vi "read RS485 subVI.vi"(8 "error in (no error)":errorcluster, 11 "VISA Refnum in":refnum<visa-resource-name>="COM5") -> (0 "error out":errorcluster, 3 "DUT Config Data":T1)   [LabVIEW 2016]
uses:
  DUT Config Data ClusterType Def.ctl
  Control 2.ctl
  <vilib>/Instr/_visa.llb/VISA Configure Serial Port (Instr).vi
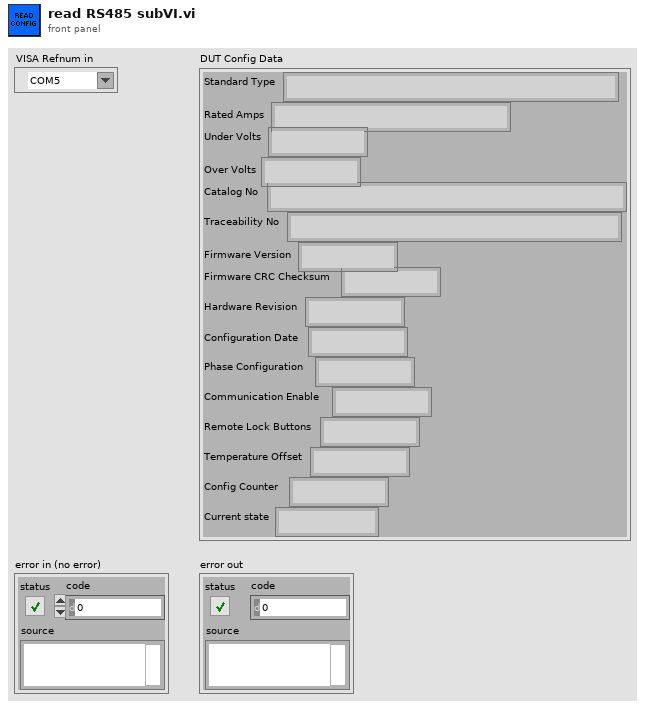
[diagram p1: front panel]
types:
  T1 = typedef "DUT Config Data ClusterType Def.ctl" = cluster{"Standard Type":string, "Rated Amps":string, "Under Volts":string, "Over Volts":string, "Catalog No":string, "Traceability No":string, "Firmware Version":string, "Firmware CRC Checksum":string, "Hardware Revision":string, "Configuration Date":string, "Phase Configuration":string, "Communication Enable":string, "Remote Lock Buttons":string, "Temperature Offset":string, "Config Counter":string, "Current state":string}
  T2 = typedef "Control 2.ctl" = enum16{"Message", "Write Config", "Read Config", "Listen"}
  T3 = cluster{"[0]":string, "[1]":string, "[2]":string, "[3]":string, "[4]":string, "[5]":string, "[6]":string, "[7]":string, "[8]":string, "[9]":string, "[10]":string, "[11]":string, "[12]":string, "[13]":string, "[14]":string, "[15]":string}
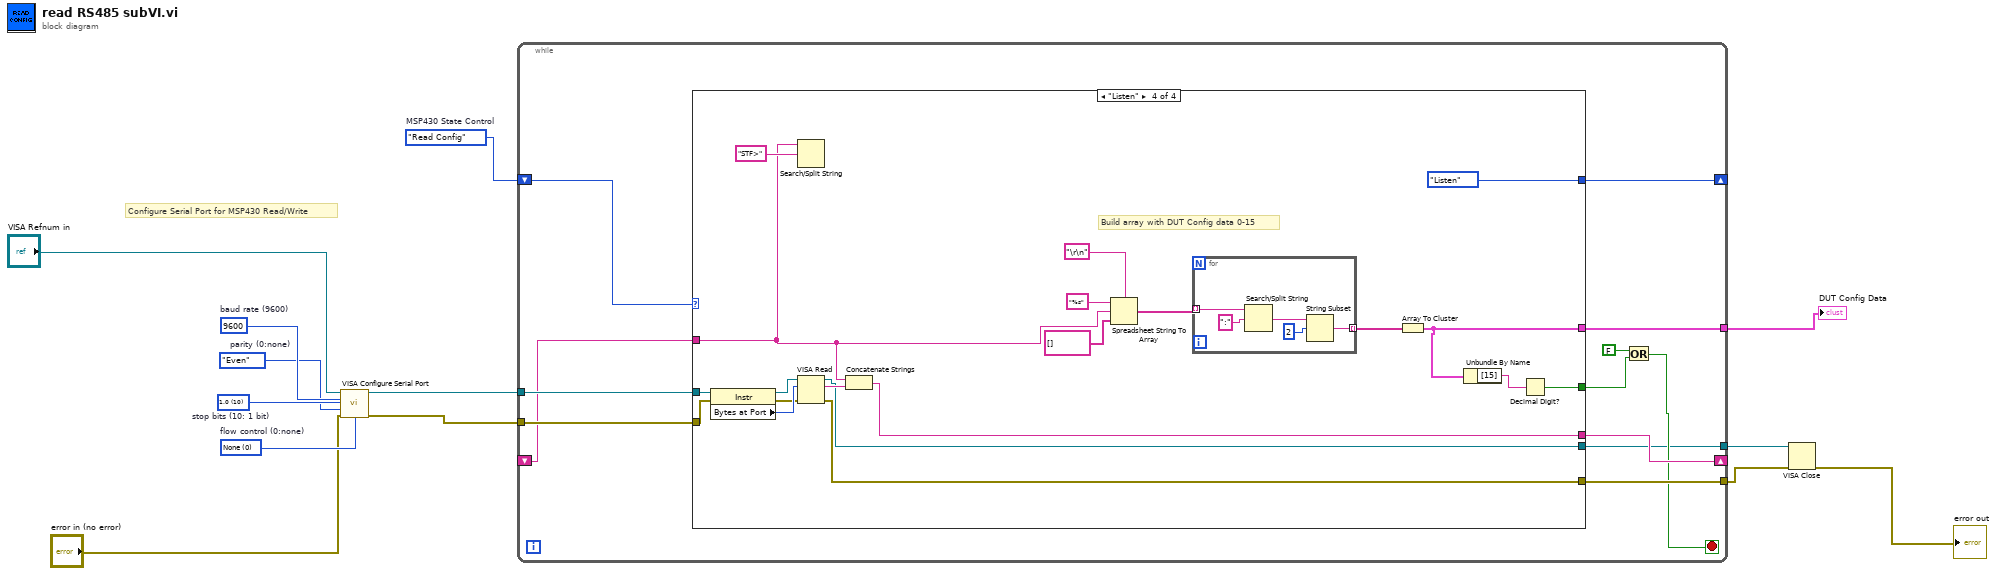
[diagram p0: block diagram]
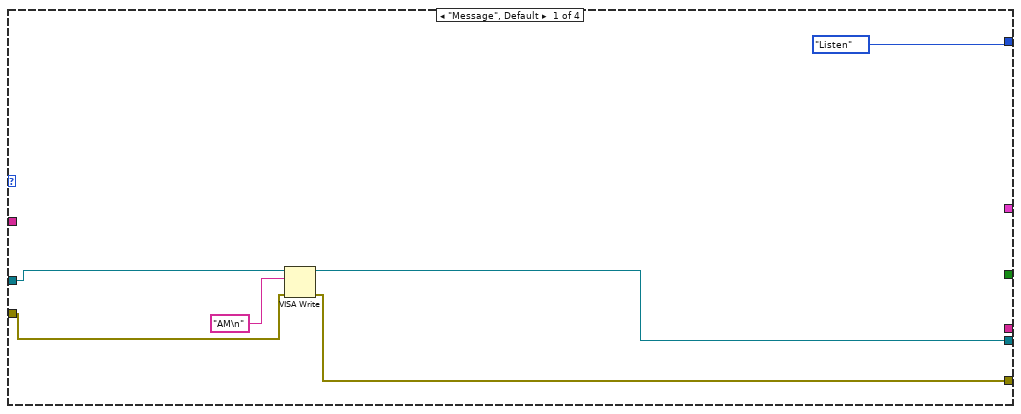
[diagram p2: hidden frame]
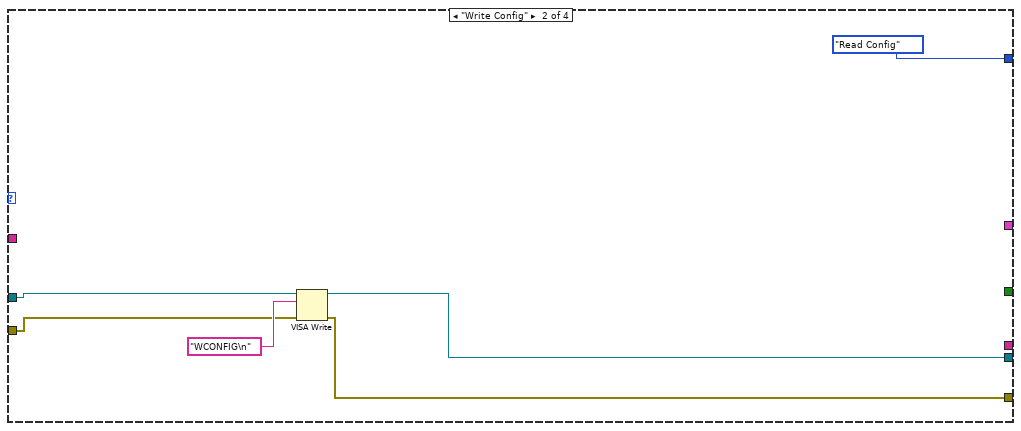
[diagram p3: hidden frame]
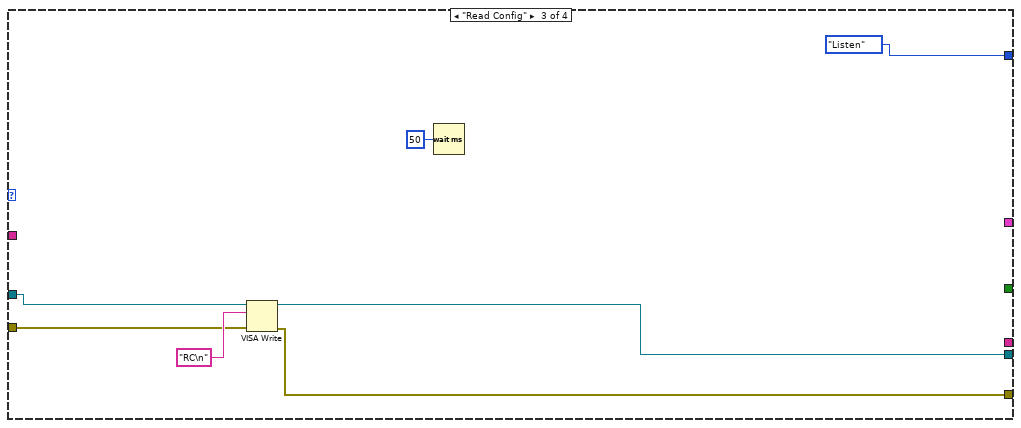
[diagram p4: hidden frame]
diagram:
  w10 = Control_2."Read Config"  # MSP430 State Control
  w7 = u16 0 items=["None", "XON/XOFF", "RTS/CTS", "XON/XOFF & RTS/CTS", "DTR/DSR", "XON/XOFF & DTR/DSR"]  # flow control (0:none)
  w6 = u16 10 items=["1.0"=10, "1.5"=15, "2.0"=20]  # stop bits (10: 1 bit)
  w5 = u32 9600  # baud rate (9600)
  w1 = enum16{"None", "Odd", "Even", "Mark", "Space"}."Even"  # parity (0:none)
  # "Configure Serial Port for MSP430 Read/Write"
  n1 = call-poly "VISA Configure Serial Port"("VISA resource name"="VISA Refnum in", "baud rate (9600)"=w5, "parity (0:none)"=w1, "error in (no error)"="error in (no error)", "stop bits (10: 1 bit)"=w6, "flow control (0:none)"=w7) -> ("VISA resource name out"=w3:refnum<visa-resource-name>, "error out"=w4:errorcluster)  [unwired: 8 in]
  n2 = while {
    tunnel: w3 -> [w25]
    tunnel: w4 -> [w24]
    shift-right: [w23] -> _
    shift-left: _ -> [w16]
    tunnel: [w22] -> w8
    shift-right: [w21] -> _
    shift-left: w10 -> [w20]
    tunnel: [w17] -> w11
    tunnel: [w14] -> w13
    stop <- w19 stop-if-true
    n3 = case shown="\"Listen\"" w20 {
      tunnel: w25 -> [w30 w36 w43 w56]
      tunnel: w24 -> [w29 w35 w42 w55]
      tunnel: [_ _ _ w53] -> w23
      tunnel: [w28 w34 w41 w52] -> w22
      tunnel: [Control_2."Listen" Control_2."Read Config" Control_2."Listen" Control_2."Listen"] -> w21
      tunnel: [_ _ _ w48] -> w18
      tunnel: [w26 w32 w38 w47] -> w17
      tunnel: w16 -> [_ _ _ w46]
      tunnel: [_ _ _ w45] -> w14
      frame "Message", Default {
        n4 = VISA Write(VISA resource name=w30, write buffer="AM\n", error in (no error)=w29) -> (VISA resource name out=w26:refnum<visa-resource-name>, error out=w28:errorcluster)  [unwired: 1 out]
      }
      frame "Write Config" {
        n5 = VISA Write(VISA resource name=w36, write buffer="WCONFIG\n", error in (no error)=w35) -> (VISA resource name out=w32:refnum<visa-resource-name>, error out=w34:errorcluster)  [unwired: 1 out]
      }
      frame "Read Config" {
        n6 = VISA Write(VISA resource name=w43, write buffer="RC\n", error in (no error)=w42) -> (VISA resource name out=w38:refnum<visa-resource-name>, error out=w41:errorcluster)  [unwired: 1 out]
        n7 = Wait (ms)(milliseconds to wait=u32 50) -> ()  [unwired: 1 out]
      }
      frame "Listen" {
        # "Build array with DUT Config data 0-15"
        n8 = property class="Instr"(reference=w56, error in=w55) -> (reference out=w57:refnum<visa-resource-name>, error out=w58:errorcluster, "Bytes at Port"=w62:u32)
        n9 = Search/Split String(string=w46, search string/char (-)="STF>") -> ()  [unwired: 1 in, 3 out]
        n10 = VISA Read(VISA resource name=w57, byte count=w62, error in (no error)=w58) -> (VISA resource name out=w47:refnum<visa-resource-name>, read buffer=w63:string, error out=w52:errorcluster)  [unwired: 1 out]
        n11 = Concatenate Strings(w46, w63) -> (w53:string)
        n12 = Spreadsheet String To Array(delimiter (Tab)="\r\n", format string="%s", spreadsheet string=w46, array type (2D Dbl)=string[] []) -> (array=w54:string[])
        n13 = for {
          tunnel: w54 -> [w69] mode=indexing
          tunnel: [w65] -> w50 mode=indexing
          n14 = Search/Split String(string=w69, search string/char (-)=":") -> (match + rest of string=w67:string)  [unwired: 1 in, 2 out]
          n15 = String Subset(string=w67, offset (0)=2) -> (substring=w65:string)  [unwired: 1 in]
        }
        n16 = Array To Cluster(array=w50) -> (cluster=w45:T3)
        n17 = Unbundle By Name(w45) -> ("[15]"=w49:string)
        n18 = Decimal Digit?(1:w49) -> (0:w48:bool)
      }
    }
    n19 = Or(x=FALSE, y=w18) -> (x .or. y?=w19:bool)
  }
  "DUT Config Data" <- w13
  n20 = VISA Close(VISA resource name=w11, error in (no error)=w8) -> (error out=→"error out":errorcluster)
